vi "Roboteq Loop.vi"(8 "error in":errorcluster) -> (0 "error out":errorcluster)   [LabVIEW 2012]
uses:
  <vilib>/Platform/TimedLoop/XDataNode/timing_clust.ctl
  <vilib>/Platform/TimedLoop/XDataNode/nitl_modes.ctl
  <vilib>/Platform/TimedLoop/XDataNode/wakeup.ctl
  Utilities/Robot Parameters/Robot Parameters.vi
  <vilib>/robotics/Steering/Steering Frame/Apply Steering Frame Velocity to Motors.vi
  Public/Set RPM.vi
  <vilib>/Platform/TimedLoop/XDataNode/XDataNode.xnode
  <vilib>/Platform/TimedLoop/XDataNode/XDNodeRunTimeDep.lvlib
  <vilib>/robotics/Steering/Steering Frame/NI_Robotics_Steering Frame.lvclass
  Roboteq.lvlib
panel:
  out "Telemetry":T1={"Voltage"={0.0, 0.0, 0.0}, "Encoder Speed"={0, 0}, "Temps"={"IC Temp (C)"=0, "Ch1 Temp (C)"=0, "Ch2 Temp (C)"=0}, "Current"={0.0, 0.0, 0.0, 4.6238981750249924e+36}} {"Current" scale=0.0..16.0; "Temps"."IC Temp (C)" scale=0.0..150.0; "Temps"."Ch1 Temp (C)" scale=0.0..150.0; "Temps"."Ch2 Temp (C)" scale=0.0..150.0; "Encoder Speed" scale=-100.0..100.0; "Voltage" scale=8.0..14.0}
  in  "VISA resource name":refnum<visa-resource-name>
  in  "Debug":bool
  out "Command to Serial":string
  in  "stop?":bool
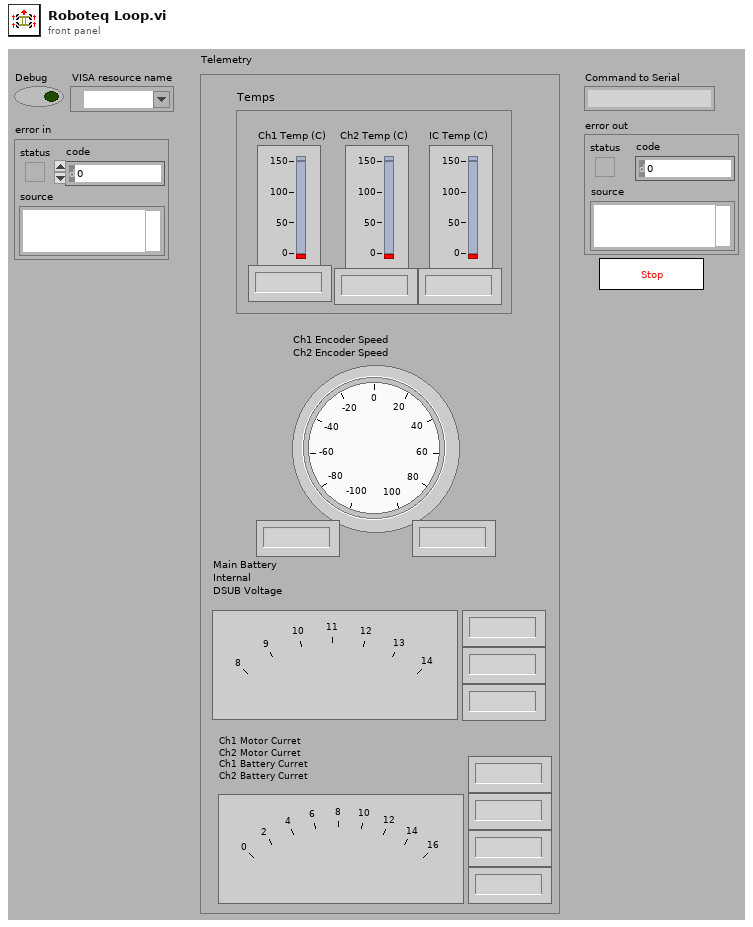
[diagram p1: front panel]
types:
  T1 = cluster{"Voltage":cluster{sgl, sgl, sgl}, "Encoder Speed":cluster{i32, i32}, "Temps":cluster{"IC Temp (C)":i32, "Ch1 Temp (C)":i32, "Ch2 Temp (C)":i32}, "Current":cluster{dbl, dbl, dbl, dbl}}
  T2 = typedef "XDNodeRunTimeDep.lvlib/timing_clust.ctl" = cluster{"Expected End [f-1]":u64, "Actual End [f-1]":u64, "Finished Late? [f-1]":bool, "Expected End [i-1]":u64, "Actual End [i-1]":u64, "Finished Late? [i-1]":bool, "Expected Start [i]":u64, "Actual Start [i]":u64, "Expected Start [f]":u64, "Actual Start [f]":u64, "Source Name":string, "Structure Name":string, "Period":i64, "Deadline":i64, "Offset":i64, "Start":i64, "Priority":i32, "Timeout":i32, "Mode":T3, "Wakeup Reason":T4, "Error":errorcluster, "Source Type":string, "Secondary Source Type":string, "Global End Time":u64, "Global Start Time":u64, "Frame Duration":u64, "Iteration Duration":u64, "Assigned CPU":i32, "I/O Scan Engine Mode":u32}
  T3 = typedef "XDNodeRunTimeDep.lvlib/nitl_modes.ctl" = enum32{"No Change", "Process missed periods, maintain original phase", "Discard missed periods, maintain original phase", "Process missed periods, ignore original phase", "Discard missed periods, ignore original phase"}
  T4 = typedef "XDNodeRunTimeDep.lvlib/wakeup.ctl" = enum32{"Normal", "Aborted", "Asynchronous wakeup", "Timing source error", "Timed loop error", "Timeout"}
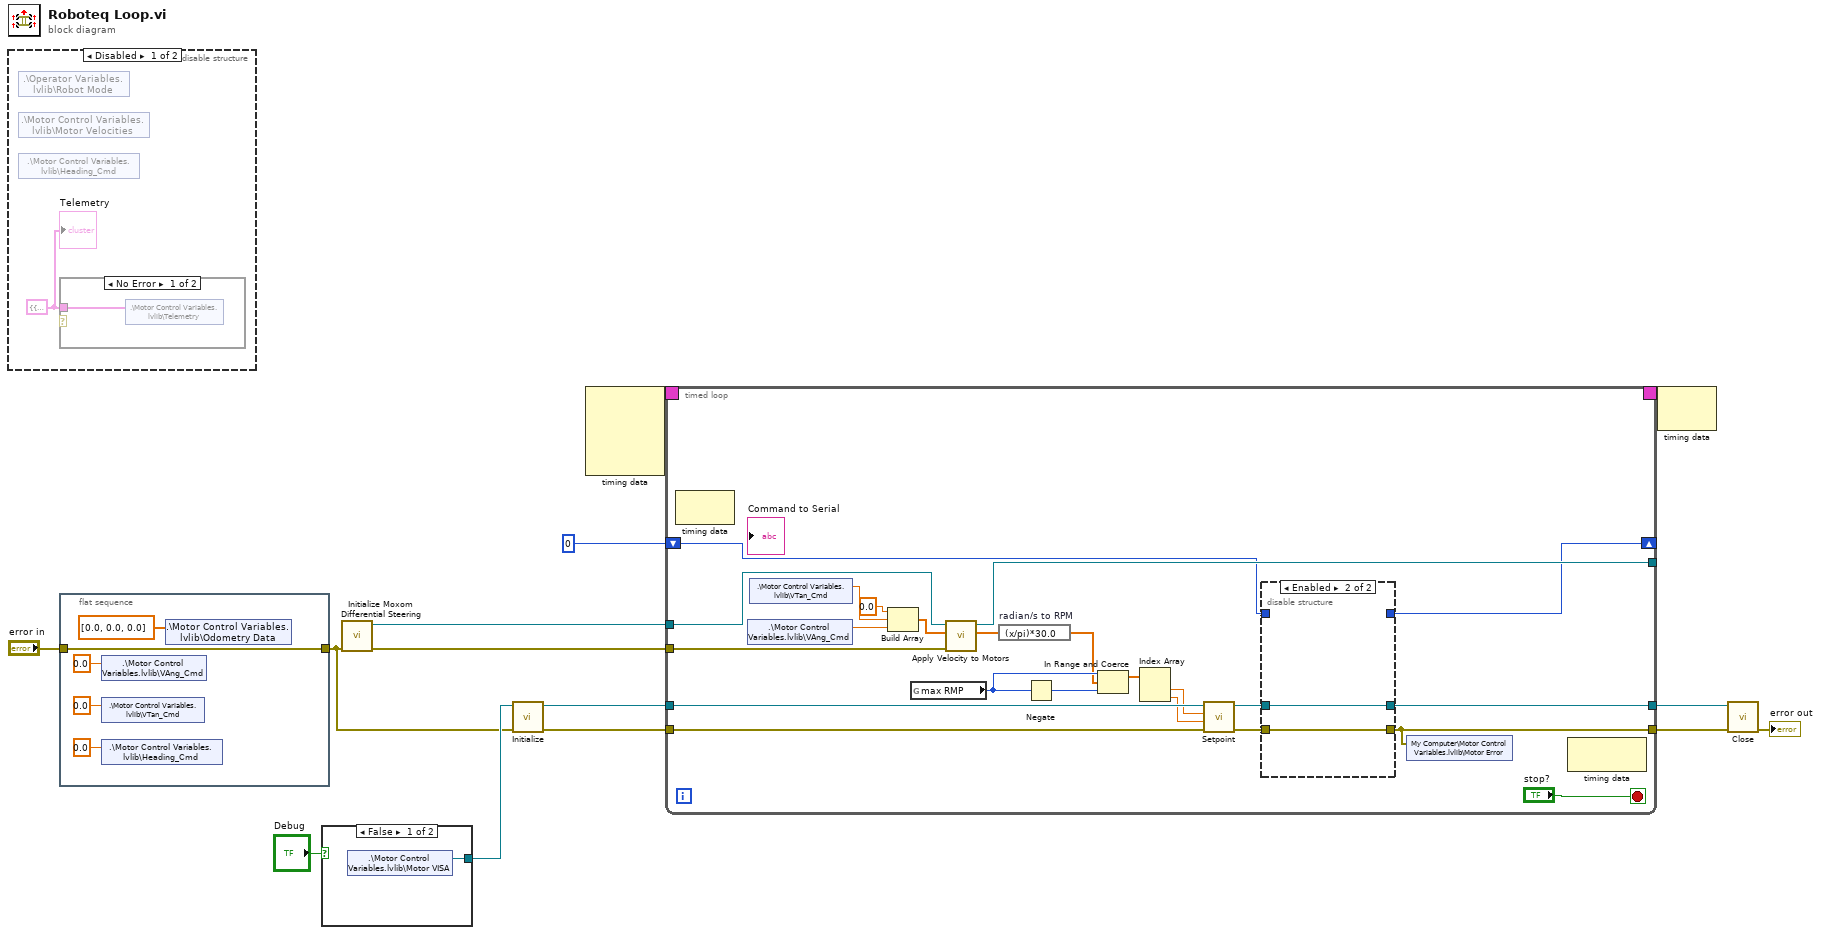
[diagram p0: block diagram]
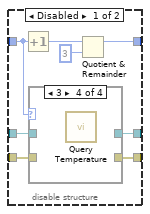
[diagram p4: hidden frame]
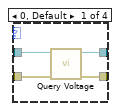
[diagram p5: hidden frame]
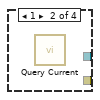
[diagram p6: hidden frame]
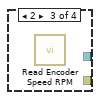
[diagram p7: hidden frame]
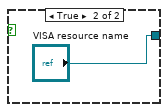
[diagram p8: hidden frame]
diagram:
  n1 = disable-structure shown="Disabled" {
    frame Disabled {
      w15 = T1 {"Voltage"={0.0, 0.0, 0.0}, "Encoder Speed"={0, 0}, "Temps"={"IC Temp (C)"=0, "Ch1 Temp (C)"=0, "Ch2 Temp (C)"=0}, "Current"={0.0, 0.0, 0.0, 0.0}} ("Telemetry")
      n2 = shared-variable ".\\Operator Variables.lvlib\\Robot Mode"() -> ()  [unwired: 1 in, 2 out]
      n3 = shared-variable ".\\Motor Control Variables.lvlib\\Motor Velocities"() -> ()  [unwired: 2 in, 1 out]
      n4 = shared-variable ".\\Motor Control Variables.lvlib\\Heading_Cmd"() -> ()  [unwired: 1 in, 2 out]
      n5 = case shown="No Error" {
        selector: _ -> [_ _]
        tunnel: w15 -> [w16 _]
        frame No Error {
          n6 = shared-variable ".\\Motor Control Variables.lvlib\\Telemetry"(w16) -> ()  [unwired: 1 in, 1 out]
        }
        frame Error {
        }
      }
      "Telemetry" <- w15
    }
    frame Enabled {
    }
  }
  n7 = flat-sequence {
    tunnel: [w17] -> w7
    tunnel: "error in" -> [w17]
    frame #0 {
      n8 = shared-variable ".\\Motor Control Variables.lvlib\\VAng_Cmd"(0.0 ("VX_Cmd")) -> ()  [unwired: 1 in, 1 out]
      n9 = shared-variable ".\\Motor Control Variables.lvlib\\VTan_Cmd"(0.0 ("VY_Cmd")) -> ()  [unwired: 1 in, 1 out]
      n10 = shared-variable ".\\Motor Control Variables.lvlib\\Heading_Cmd"(0.0 ("Heading_Cmd")) -> ()  [unwired: 1 in, 1 out]
      n11 = shared-variable ".\\Motor Control Variables.lvlib\\Odometry Data"(dbl[] [0.0, 0.0, 0.0] ("Odometry Data")) -> ()  [unwired: 1 in, 1 out]
    }
  }
  n12 = case shown="False" "Debug" {
    tunnel: [w22 "VISA resource name"] -> w8
    frame False {
      n13 = shared-variable ".\\Motor Control Variables.lvlib\\Motor VISA"() -> (w22:refnum<visa-resource-name>)  [unwired: 1 in, 1 out]
    }
    frame True {
    }
  }
  n14 = call "Initialize Moxom Differential Steering.vi"("error in (no error)"=w7) -> ("error out"=w9:errorcluster, "differential steering frame out"=w10:refnum<class "NI_Robotics_Differential Steering Frame.lvclass">)  [unwired: 9 in]
  n15 = call "Initialize.vi"("error in (no error)"=w7, "VISA resource name"=w8) -> ("error out"=w5:errorcluster, "VISA resource name out"=w6:refnum<visa-resource-name>)  [unwired: 8 in]
  n16 = node-c288() -> (w12:T2)  [unwired: 4 in]
  n17 = timed-loop {
    timing: w12 -> [_]
    timing-out: [_] -> w11
    tunnel: w10 -> [w45]
    tunnel: w9 -> [w46]
    tunnel: [w40] -> _
    tunnel: w6 -> [w34]
    tunnel: w5 -> [w33]
    shift-right: [w26] -> _
    shift-left: 0 -> [w27]
    tunnel: [w28] -> w3
    tunnel: [w24] -> w2
    stop <- "stop?" stop-if-true
    n18 = node-c288() -> ()  [unwired: 1 in, 1 out]
    n19 = shared-variable ".\\Motor Control Variables.lvlib\\VAng_Cmd"() -> (w42:dbl)  [unwired: 1 in, 1 out]
    n20 = shared-variable ".\\Motor Control Variables.lvlib\\VTan_Cmd"() -> (w43:dbl)  [unwired: 1 in, 1 out]
    n21 = Build Array(0.0 ("element"), w43, w42) -> (w41:dbl[])
    n22 = global read "Robot Parameters.vi" "max RMP"() -> (w37:i32)
    n23 = call-poly <vilib>:"Apply Velocity to Motors.vi"("error in (no error)"=w46, "steering frame velocity"=w41, "steering frame in"=w45) -> ("ccw motor velocity setpoints"=w39:dbl[], "steering frame out"=w40:refnum<class "NI_Robotics_Differential Steering Frame.lvclass">)  [unwired: 4 in, 3 out]
    n24 = expression code="(x/pi)*30.0" "radian/s to RPM"(w39) -> (w36:dbl[])
    n25 = Negate(x=w37) -> (-x=w38:i32)
    n26 = In Range and Coerce(upper limit=w37, x=w36, lower limit=w38) -> (coerced(x)=w35:dbl[])  [unwired: 1 out]
    n27 = Index Array(array=w35) -> (element #1=w32:dbl, element #2=w31:dbl)  [unwired: 2 in]
    n28 = call-poly "Setpoint.vi"("error in (no error)"=w33, "Motor2 Speed (RPM)"=w31, "Motor1 Speed (RPM)"=w32, "VISA resource name"=w34) -> ("error out"=w29:errorcluster, "VISA resource name out"=w30:refnum<visa-resource-name>)  [unwired: 5 in, 1 out]
    n29 = disable-structure shown="Enabled" {
      disable-tunnel: w30 -> [w54 w60]
      disable-tunnel: w29 -> [w53 w59]
      disable-tunnel: [w52 w60] -> w28
      disable-tunnel: [w51 w59] -> w24
      disable-tunnel: w27 -> [w50 _]
      disable-tunnel: [w47 _] -> w26
      frame Disabled {
        n30 = Increment(x=w50) -> (x+1=w49:i32)
        n31 = case shown="3" w50 {
          tunnel: w54 -> [w58 _ _ _]
          tunnel: w53 -> [w57 _ _ _]
          tunnel: [w56 _ _ _] -> w52
          tunnel: [w55 _ _ _] -> w51
          frame 0, Default {
            n32 = call "Query Voltage.vi"("error in (no error)"=w57, "VISA resource name"=w58) -> ("error out"=w55:errorcluster, "VISA resource name out"=w56:refnum<visa-resource-name>)  [unwired: 4 in, 4 out]
          }
          frame 1 {
            n33 = call "Query Current.vi"() -> ()  [unwired: 5 in, 7 out]
          }
          frame 2 {
            n34 = call "Read Encoder Speed RPM.vi"() -> ()  [unwired: 9 in, 3 out]
          }
          frame 3 {
            n35 = call "Query Temperature.vi"() -> ()  [unwired: 6 in, 6 out]
          }
        }
        n36 = Quotient & Remainder(x=w49, y=3) -> (x-y*floor(x/y)=w47:i32)  [unwired: 1 out]
      }
      frame Enabled {
      }
    }
    n37 = shared-variable "My Computer\\Motor Control Variables.lvlib\\Motor Error"(w24) -> ()  [unwired: 1 in, 1 out]
    n38 = node-c288() -> ()  [unwired: 1 in, 1 out]
  }
  n39 = node-c288(w11) -> ()  [unwired: 1 out]
  n40 = call "Close.vi"("error in (no error)"=w2, "VISA resource name"=w3) -> ("error out"=→"error out":errorcluster)  [unwired: 9 in]
